vi "Start Generator.vi"(7 "Timeout ms":i32=500, 8 "error in (no error)":errorcluster, 11 "Wrapper in":refnum<class "Wrapper.lvclass">) -> (0 "error out":errorcluster, 2 "New Message Event":refnum<user-event>, 3 "Wrapper out":refnum<class "Wrapper.lvclass">)   [LabVIEW 2020, in "Wrapped Actor.lvlib" / "Wrapper.lvclass"]
uses:
  Wrapper.lvclass
  <vilib>/ActorFramework/Message/Message.lvclass
  Generator/Generator.lvclass
  C:/Program Files/National Instruments/LabVIEW 2020/vi.lib/ActorFramework/Actor/Actor.lvclass
  Actor Pub Sub Channels/Pub Sub Event Channel/Pub Sub Event Channel.lvclass
  E:/Labview/LV 2020/Libs/Actor Pub Sub/Source/Actor Pub Sub Channels/Pub Sub Message Channel/Pub Sub Message Channel.lvclass
  Actor Pub Sub Channels/Pub Sub Event Channel/Pub Sub Event Channel.lvclass/Pub Sub Event Channel.ctl
  Generator/Generator.lvclass/Generator.ctl
  Wrapper.lvclass/Wrapper.ctl
  Generator/Write Result Receiver.vi
  Generator/Write Timeout ms.vi
  Actor Pub Sub Channels/Pub Sub Event Channel/Read New Message Event.vi
  Actor Pub Sub Channels/Pub Sub Message Channel/Pub Sub Message Channel.lvclass
  <vilib>/ActorFramework/Actor/Actor.lvclass
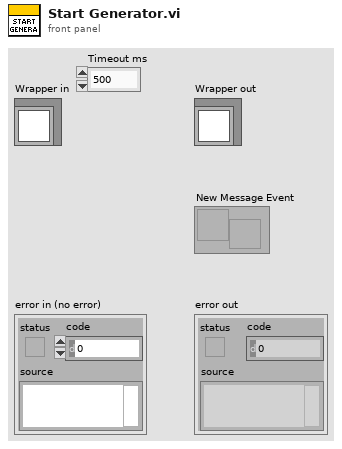
[diagram p1: front panel]
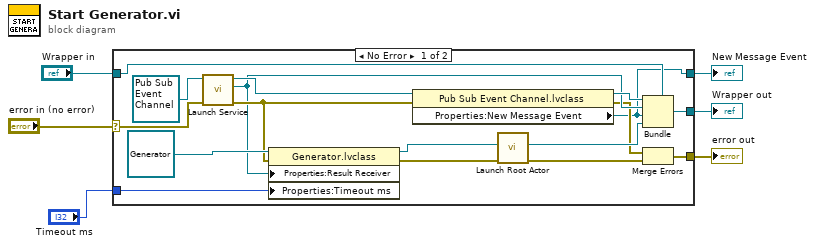
[diagram p0: block diagram]
diagram:
  n1 = case shown="No Error" "error in (no error)" {
    selector: "error in (no error)" -> [w12 w25]
    tunnel: [w9 w25] -> w5
    tunnel: [w18 w24] -> w3
    tunnel: "Wrapper in" -> [w23 w24]
    tunnel: [w8 _] -> w2
    tunnel: "Timeout ms" -> [w7 _]
    frame No Error {
      n2 = call "Launch Service.vi"("error in (no error)"=w12, "Pub Sub Message Channel"=refnum<class "Pub Sub Event Channel.lvclass"> refnum ("Actor Pub Sub Channels.lvlib:Pub Sub Event Channel.lvclass")) -> ("error out"=w19:errorcluster, "Enqueuer"=w16:refnum<class "Message Enqueuer.lvclass">, "Pub Sub Message Channel Out"=w20:refnum<class "Pub Sub Event Channel.lvclass">)  [unwired: 7 in]
      n3 = property class="Generator.lvclass"(reference=refnum<class "Generator.lvclass"> refnum ("Wrapped Actor.lvlib:Generator.lvclass"), error in=w19, "Properties:Result Receiver"=w16, "Properties:Timeout ms"=w7) -> (reference out=w14:refnum<class "Generator.lvclass">, error out=w15:errorcluster)
      n4 = property class="Pub Sub Event Channel.lvclass"(reference=w20, error in=w19) -> (reference out=w17:refnum<class "Pub Sub Event Channel.lvclass">, error out=w10:errorcluster, "Properties:New Message Event"=w8:refnum<user-event>)
      n5 = call <vilib>:"Launch Root Actor.vi"("error in (no error)"=w15, "Actor"=w14) -> ("error out"=w11:errorcluster, "Actor's Enqueuer"=w13:refnum<class "Message Enqueuer.lvclass">)  [unwired: 8 in]
      n6 = Bundle(cluster=w23, w17, w16, w8, w13) -> (w18:refnum<class "Wrapper.lvclass">)
      n7 = Merge Errors(w10, w11) -> (w9:errorcluster)
    }
    frame Error {
    }
  }
  "error out" <- w5
  "Wrapper out" <- w3
  "New Message Event" <- w2
